vi "Timed Loop Time.vi"(8 "error in (no error)":errorcluster, 10 "ET since start (s)":dbl, 11 "State in":T1={"State"=enum."Idle", "Start Time"=timestamp(0 s since 1904-01-01), "Configuration"={"Cycle Period"=0.0, "Bronkhorst M13"={"VISA resource name"="", "Simulated?"=FALSE}, "Flow Meter Type"="", "Bronkhorst M14"={"VISA resource name"="", "Simulated?"=FALSE}}, "Current Time"=timestamp(0 s since 1904-01-01), "First Iteration"=FALSE, "Data"={"Flow Meter Read(g/min)"=0.0}, "Process Name"=""}) -> (0 "error out":errorcluster, 3 "State out":T1={"State"=enum."Idle", "Start Time"=timestamp(0 s since 1904-01-01), "Configuration"={"Cycle Period"=0.0, "Bronkhorst M13"={"VISA resource name"="", "Simulated?"=FALSE}, "Flow Meter Type"="", "Bronkhorst M14"={"VISA resource name"="", "Simulated?"=FALSE}}, "Current Time"=timestamp(0 s since 1904-01-01), "First Iteration"=FALSE, "Data"={"Flow Meter Read(g/min)"=0.0}, "Process Name"=""})   [LabVIEW 2018, in "Flow Module.lvlib" / "Flow Module Engine.lvlib"]
uses:
  Flow Module Engine.lvlib
  State Cluster.ctl
  State Enum.ctl
  Feed Module/Controls/Flow Module Settings Cluster.ctl
  Mettler Toledo/Controls/Settings Cluster.ctl
  Flow Module.lvlib
  Mettler Toledo/Mettler Toledo.lvlib
panel:
  # "Flow Meter Settings"
  # "Flow Meter Settings"
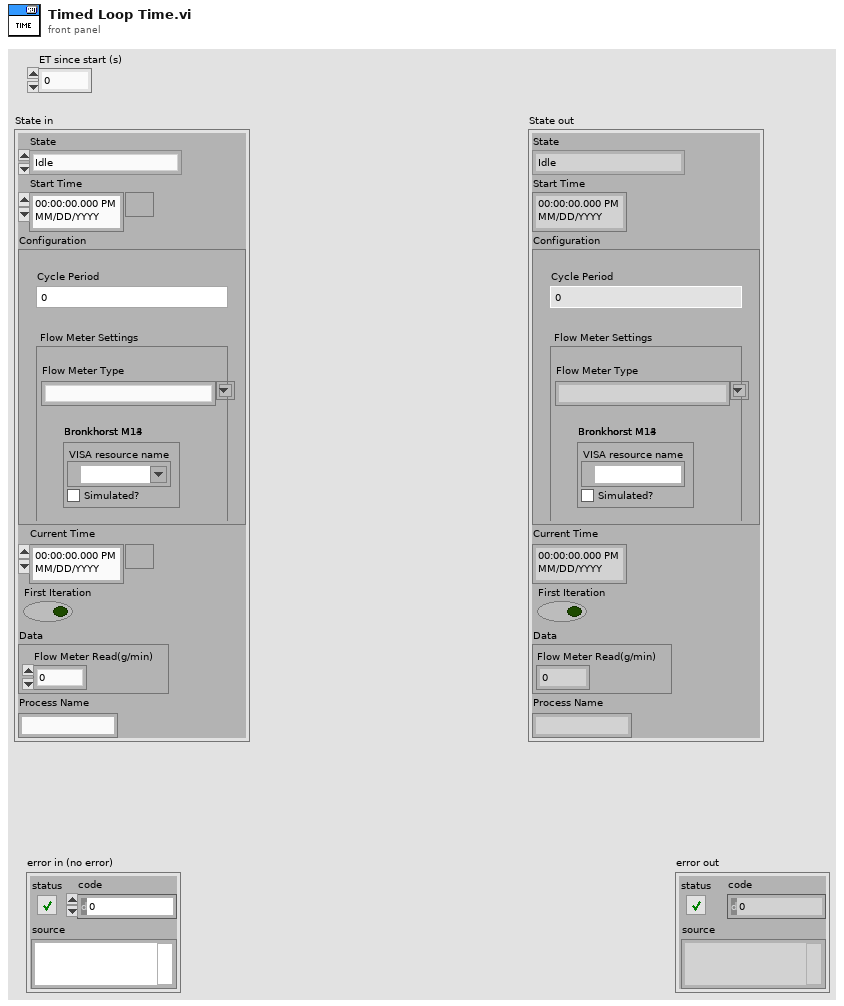
[diagram p1: front panel]
types:
  T1 = typedef "Flow Module.lvlib/Flow Module Engine.lvlib/State Cluster.ctl" = cluster{"State":T2, "Start Time":timestamp, "Configuration":T3, "Current Time":timestamp, "First Iteration":bool, "Data":cluster{"Flow Meter Read(g/min)":dbl}, "Process Name":string}
  T2 = typedef "Flow Module.lvlib/Flow Module Engine.lvlib/State Enum.ctl" = enum16{"Measuring", "Idle"}
  T3 = typedef "Flow Module.lvlib/Flow Module Settings Cluster.ctl" = cluster{"Cycle Period":dbl, "Bronkhorst M13":T4, "Flow Meter Type":string, "Bronkhorst M14":T4}
  T4 = typedef "Mettler Toledo.lvlib/Settings Cluster.ctl" = cluster{"VISA resource name":refnum<visa-resource-name>, "Simulated?":bool}
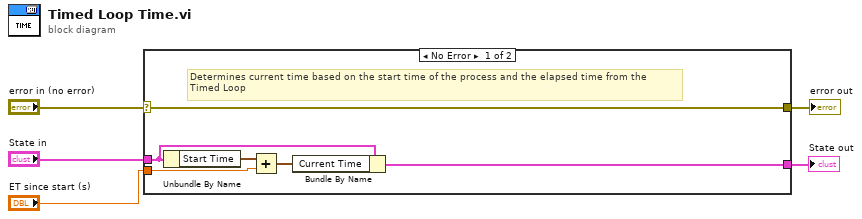
[diagram p0: block diagram]
diagram:
  n1 = case shown="No Error" "error in (no error)" {
    selector: "error in (no error)" -> [w6 w13]
    tunnel: [w6 w13] -> w4
    tunnel: "State in" -> [w11 w12]
    tunnel: [w10 w12] -> w2
    tunnel: "ET since start (s)" -> [w8 _]
    frame No Error {
      # "Determines current time based on the start time of the process and the elapsed time from the\nTimed Loop"
      n2 = Unbundle By Name(w11) -> ("Start Time"=w9:timestamp)
      n3 = Add(x=w9, y=w8) -> (x+y=w7:timestamp)
      n4 = Bundle By Name(cluster=w11, "Current Time"=w7) -> (w10:T1)
    }
    frame Error {
    }
  }
  "error out" <- w4
  "State out" <- w2
